vi "standalone resonant correction.vi"(0 "uncorrected images in":i16[][][](array[numeric]), 2 "force reset shift registers":bool, 7 "frames.p.queue.item":dbl, 9 "x.pixels":dbl, 11 "y.pixels":dbl, 13 "no.of.channels":dbl) -> (4 "corrected images out":i16[][][](array[numeric]))   [LabVIEW 2012]
doc: "SciScan 1.2 160622"
uses:
  GFG/GFGbooleanGet.vi
  GFG/GFGnumericGet.vi
  GFG/GFG library.lvlib
panel:
  in  "image probe on":bool
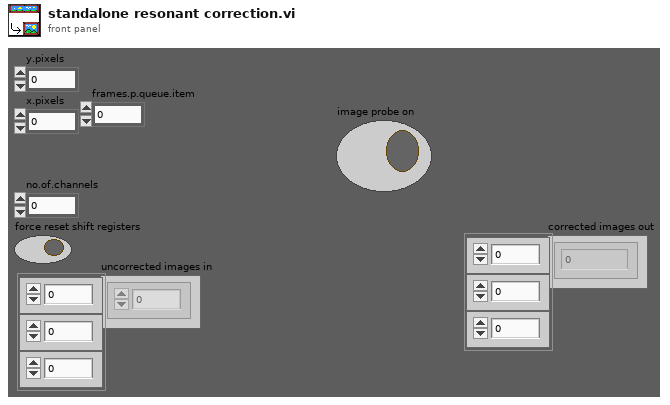
[diagram p1: front panel]
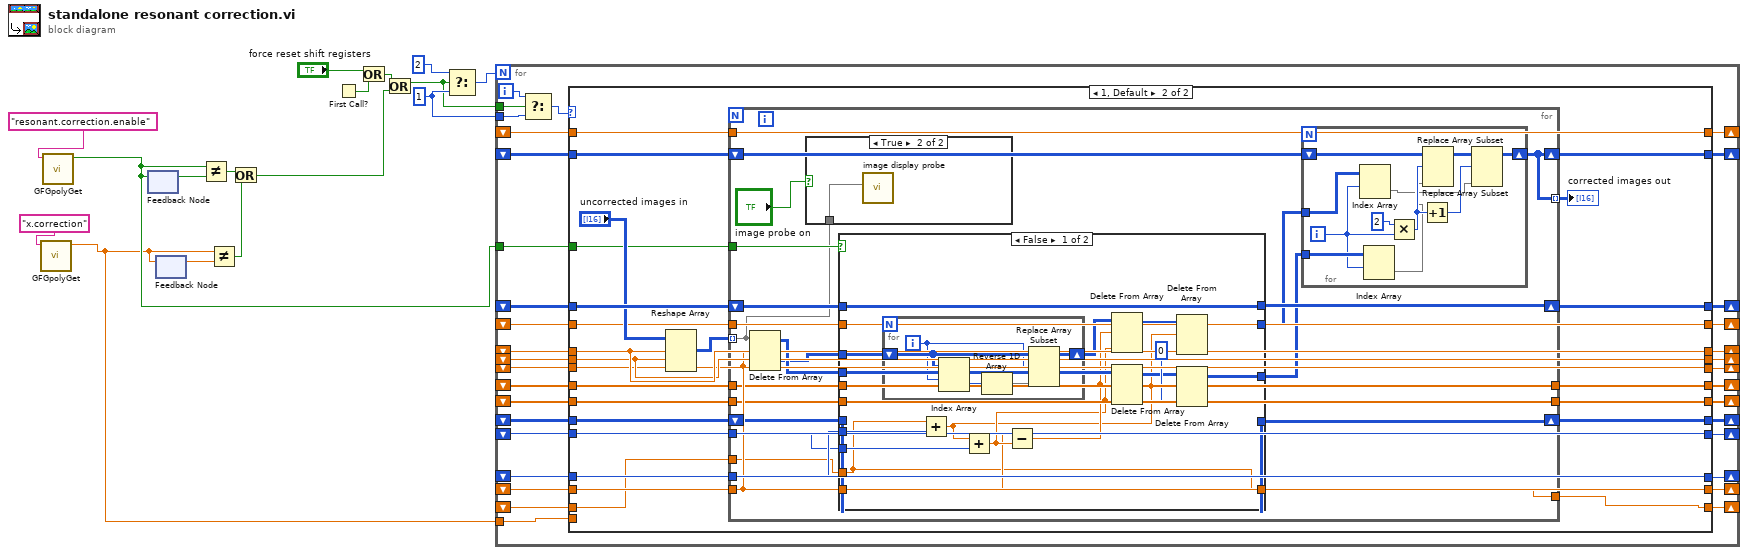
[diagram p0: block diagram]
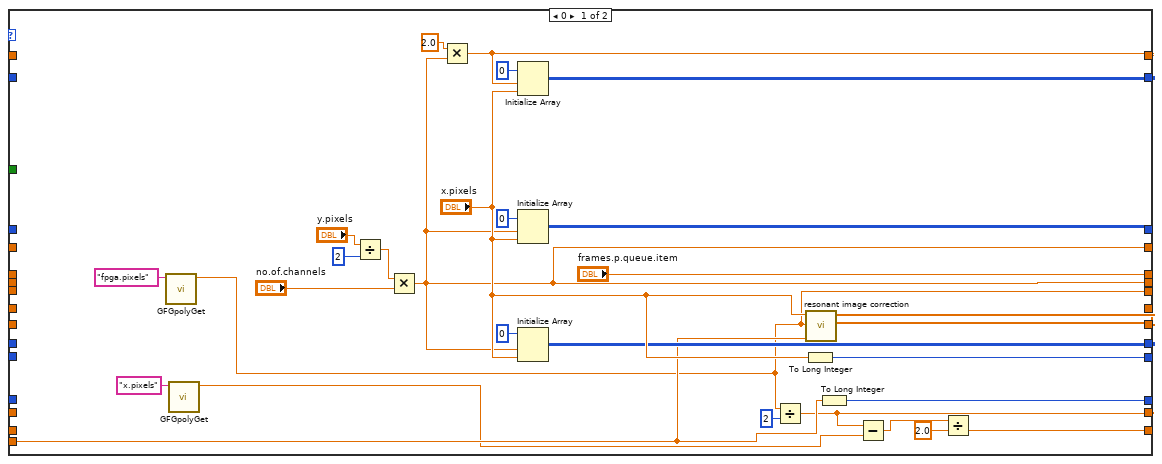
[diagram p2: hidden frame]
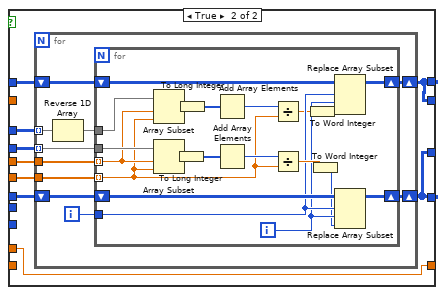
[diagram p4: hidden frame]
diagram:
  w11 = i16 1 ("sum")
  n1 = call-poly "GFGpolyGet.vi"("Variable Name in"="x.correction" ("Tag in")) -> ("Numeric"=w1:dbl)  [unwired: 8 in, 2 out]
  n2 = call-poly "GFGpolyGet.vi"("Variable Name in"="resonant.correction.enable" ("Tag in")) -> ("Boolean Value OUT"=w2:bool)  [unwired: 9 in, 1 out]
  n3 = feedback #1() -> (w6:bool)  [unwired: 1 in]
  n4 = feedback-in #1(w2) -> ()
  n5 = feedback #2() -> (w9:dbl)  [unwired: 1 in]
  n6 = feedback-in #2(w1) -> ()
  n7 = Not Equal?(x=w2, y=w6) -> (x != y?=w7:bool)
  n8 = Not Equal?(x=w1, y=w9) -> (x != y?=w10:bool)
  n9 = Or(x=w7, y=w10) -> (x .or. y?=w3:bool)
  n10 = First Call?() -> (First Call?: T/F=w15:bool)
  n11 = Or(x="force reset shift registers", y=w15) -> (x .or. y?=w12:bool)
  n12 = Or(x=w12, y=w3) -> (x .or. y?=w4:bool)
  n13 = Select(t=i16 2 ("sum"), s=w4, f=w11) -> (s? t:f=w13:i16)
  n14 = for {
    N: w13 -> [_]
    shift-right: [w42] -> _
    shift-left: _ -> [w48]
    shift-right: [w43] -> _
    shift-left: _ -> [w47]
    shift-right: [w36] -> _
    shift-left: _ -> [w37]
    shift-right: [w34] -> _
    shift-left: _ -> [w46]
    shift-right: [w33] -> _
    shift-left: _ -> [w45]
    shift-right: [w31] -> _
    shift-left: _ -> [w35]
    shift-right: [w29] -> _
    shift-left: _ -> [w38]
    shift-right: [w28] -> _
    shift-left: _ -> [w40]
    shift-right: [w26] -> _
    shift-left: _ -> [w50]
    shift-right: [w27] -> _
    shift-left: _ -> [w39]
    shift-right: [w30] -> _
    shift-left: _ -> [w41]
    shift-right: [w25] -> _
    shift-left: _ -> [w44]
    shift-right: [w32] -> _
    shift-left: _ -> [w49]
    tunnel: w4 -> [w23]
    tunnel: w11 -> [w22]
    tunnel: w2 -> [w20]
    tunnel: w1 -> [w19]
    shift-right: [w18] -> _
    shift-left: _ -> [w17]
    i -> [w24]
    n15 = Select(t=w24, s=w23, f=w22) -> (s? t:f=w21:i32)
    n16 = case shown="1, Default" w21 {
      tunnel: w50 -> [_ w83]
      tunnel: w49 -> [_ w90]
      tunnel: w20 -> [_ w82]
      tunnel: w48 -> [_ w103]
      tunnel: w47 -> [_ w102]
      tunnel: w46 -> [_ w101]
      tunnel: w45 -> [_ w100]
      tunnel: w44 -> [_ w87]
      tunnel: [w63 w99] -> w43
      tunnel: [w68 w98] -> w42
      tunnel: w41 -> [_ w88]
      tunnel: w40 -> [_ w85]
      tunnel: w39 -> [_ w84]
      tunnel: w38 -> [_ w86]
      tunnel: w37 -> [_ w97]
      tunnel: [w69 w96] -> w36
      tunnel: w35 -> [_ w89]
      tunnel: [w64 w92] -> w34
      tunnel: [w65 w91] -> w33
      tunnel: [w55 w90] -> w32
      tunnel: [w70 w89] -> w31
      tunnel: [w62 w88] -> w30
      tunnel: [w60 w86] -> w29
      tunnel: ["frames.p.queue.item" w85] -> w28
      tunnel: [w60 w84] -> w27
      tunnel: [w56 w83] -> w26
      tunnel: [w61 w87] -> w25
      tunnel: w19 -> [w58 _]
      tunnel: [w53 w80] -> w18
      tunnel: w17 -> [_ w81]
      frame 0 {
        n17 = call-poly "GFGpolyGet.vi"("Variable Name in"="fpga.pixels") -> ("Numeric"=w56:dbl)  [unwired: 8 in, 2 out]
        n18 = call-poly "GFGpolyGet.vi"("Variable Name in"="x.pixels") -> ("Numeric"=w54:dbl)  [unwired: 8 in, 2 out]
        n19 = Divide(x="y.pixels", y=2) -> (x/y=w67:dbl)
        n20 = Multiply(x=w67, y="no.of.channels") -> (x*y=w60:dbl)
        n21 = Multiply(x=2.0, y=w60) -> (x*y=w70:dbl)
        n22 = Initialize Array(i16 0 ("sum"), w70, "x.pixels") -> (w69:i16[][])
        n23 = Initialize Array(i16 0 ("sum"), w60, "x.pixels") -> (w68:i16[][])
        n24 = Initialize Array(i16 0 ("sum"), w60, "x.pixels") -> (w63:i16[][])
        n25 = Divide(x=w56, y=2) -> (x/y=w55:dbl)
        n26 = To Long Integer(number="x.pixels") -> (32bit integer=w62:i32)
        n27 = call "resonant image correction.vi"("shift index"=w58, "pixels per period (2pi, 2 lines)"=w56, "x pixels"="x.pixels") -> ("histogram cumsum"=w64:dbl[], "histogram pixels to avg"=w65:dbl[])  [unwired: 7 in]
        n28 = To Long Integer(number=w58) -> (32bit integer=w61:i32)
        n29 = Subtract(x=w55, y=w54) -> (x-y=w52:dbl)
        n30 = Divide(x=w52, y=2.0) -> (x/y=w53:dbl)
      }
      frame 1, Default {
        n31 = Reshape Array("uncorrected images in", w85, w84, w83) -> (w95:i16[][][])
        n32 = for {
          tunnel: w95 -> [w107] mode=indexing
          tunnel: w90 -> [w125]
          tunnel: w82 -> [w124]
          tunnel: w101 -> [w109]
          tunnel: w100 -> [w108]
          tunnel: w87 -> [w121]
          shift-right: [w120] -> w99
          shift-left: w102 -> [w122]
          shift-right: [w119] -> w98
          shift-left: w103 -> [w123]
          tunnel: w88 -> [w118]
          tunnel: w86 -> [w117]
          shift-right: [w115] -> w96
          shift-left: w97 -> [w116]
          tunnel: w89 -> [w114]
          tunnel: [w115] -> w94 mode=indexing
          tunnel: [w109] -> w92
          tunnel: [w108] -> w91
          tunnel: w81 -> [w105]
          tunnel: [w104] -> w80
          n33 = Delete From Array(array=w107, length=w125, index (col)=w125) -> (deleted portion=w112:i16[][], array with subset deleted=w113:i16[][])  [unwired: 1 in]
          n34 = case shown="True" "image probe on" {
            tunnel: w107 -> [_ w126]
            frame False {
            }
            frame True {
              n35 = call "image display probe.vi"("Image Pixels (I16)"=w126) -> ()  [unwired: 11 in]
            }
          }
          n36 = case shown="False" w124 {
            tunnel: w112 -> [w131 w158]
            tunnel: w113 -> [w141 w157]
            tunnel: w109 -> [_ w156]
            tunnel: w108 -> [_ w155]
            tunnel: w123 -> [w142 w154]
            tunnel: w122 -> [w130 w153]
            tunnel: [w139 w150] -> w110
            tunnel: [w137 w151] -> w111
            tunnel: w121 -> [w143 _]
            tunnel: [w130 w150] -> w120
            tunnel: [w142 w151] -> w119
            tunnel: w118 -> [w136 _]
            tunnel: w117 -> [w132 _]
            tunnel: w125 -> [w128 _]
            tunnel: w105 -> [w127 w152]
            tunnel: [w127 w152] -> w104
            frame False {
              w144 = 0 ("disabled index (col)")
              n37 = for {
                N: w132 -> [_]
                shift-right: [w148] -> w129
                shift-left: w131 -> [w147]
                i -> [w146]
                n38 = Index Array(array=w147, index (row)=w146) -> (element=w145:i16[])  [unwired: 1 in]
                n39 = Reverse 1D Array(array=w145) -> (reversed array=w149:i16[])
                n40 = Replace Array Subset(array=w147, new element=w149, index (row)=w146) -> (w148:i16[][])  [unwired: 1 in]
              }
              n41 = Add(x=w127, y=w143) -> (x+y=w133:dbl)
              n42 = Add(x=w133, y=w136) -> (x+y=w134:dbl)
              n43 = Subtract(x=w128, y=w134) -> (x-y=w135:dbl)
              n44 = Delete From Array(array=w129, length=w135, index (col)=w134) -> (array with subset deleted=w138:i16[][])  [unwired: 1 in, 1 out]
              n45 = Delete From Array(array=w141, length=w135, index (col)=w134) -> (array with subset deleted=w140:i16[][])  [unwired: 1 in, 1 out]
              n46 = Delete From Array(array=w138, length=w133, index (col)=w144) -> (array with subset deleted=w137:i16[][])  [unwired: 1 in, 1 out]
              n47 = Delete From Array(array=w140, length=w133, index (col)=w144) -> (array with subset deleted=w139:i16[][])  [unwired: 1 in, 1 out]
            }
            frame True {
              n48 = for {
                tunnel: w158 -> [w166] mode=indexing
                tunnel: w157 -> [w165] mode=indexing
                tunnel: w156 -> [w168]
                tunnel: w155 -> [w167]
                shift-right: [w160] -> w151
                shift-left: w154 -> [w164]
                shift-right: [w161] -> w150
                shift-left: w153 -> [w163]
                i -> [w162]
                n49 = Reverse 1D Array(array=w166) -> (reversed array=w159:i16[])
                n50 = for {
                  tunnel: w168 -> [w187] mode=indexing
                  tunnel: w167 -> [w182] mode=indexing
                  tunnel: w159 -> [w173]
                  tunnel: w165 -> [w188]
                  shift-right: [w175] -> w160
                  shift-left: w164 -> [w179]
                  shift-right: [w176] -> w161
                  shift-left: w163 -> [w180]
                  tunnel: w162 -> [w178]
                  i -> [w174]
                  n51 = Array Subset(array=w173, index=w187, length=w182) -> (w185:i16[])
                  n52 = Array Subset(array=w188, index=w187, length=w182) -> (w186:i16[])
                  n53 = To Long Integer(number=w186) -> (32bit integer=w171:i32[])
                  n54 = To Long Integer(number=w185) -> (32bit integer=w172:i32[])
                  n55 = Add Array Elements(numeric array=w172) -> (sum=w183:i32)
                  n56 = Add Array Elements(numeric array=w171) -> (sum=w184:i32)
                  n57 = Divide(x=w183, y=w182) -> (x/y=w177:dbl)
                  n58 = Divide(x=w184, y=w182) -> (x/y=w181:dbl)
                  n59 = To Word Integer(number=w177) -> (16bit integer=w170:i16)
                  n60 = To Word Integer(number=w181) -> (16bit integer=w169:i16)
                  n61 = Replace Array Subset(array=w179, new element=w170, index (row)=w178, index (col)=w174) -> (w175:i16[][])
                  n62 = Replace Array Subset(array=w180, new element=w169, index (row)=w178, index (col)=w174) -> (w176:i16[][])
                }
              }
            }
          }
          n63 = for {
            N: w114 -> [_]
            shift-right: [w195] -> w115
            shift-left: w116 -> [w197]
            tunnel: w111 -> [w199]
            tunnel: w110 -> [w198]
            i -> [w192]
            n64 = Index Array(array=w199, index (row)=w192) -> (element=w189:i16[])  [unwired: 1 in]
            n65 = Index Array(array=w198, index (row)=w192) -> (element=w190:i16[])  [unwired: 1 in]
            n66 = Multiply(x=2, y=w192) -> (x*y=w191:i32)
            n67 = Increment(x=w191) -> (x+1=w193:i32)
            n68 = Replace Array Subset(array=w197, new element=w190, index (row)=w191) -> (w196:i16[][])  [unwired: 1 in]
            n69 = Replace Array Subset(array=w196, new element=w189, index (row)=w193) -> (w195:i16[][])  [unwired: 1 in]
          }
        }
        "corrected images out" <- w94
      }
    }
  }
